vi "Auto Drive.vi"(7 "Distance":dbl format="%#_13g", 8 "error in (no error)":errorcluster, 9 "Angle":dbl format="%#_13g", 10 "Drive":T1[](array[typedef]), 11 "Swerve":T1[](array[typedef])) -> (0 "error IO":errorcluster)   [LabVIEW 2016]
uses:
  <vilib>/Rock Robotics/WPI/MotorControl/WPI_MotorControlDeviceRef.ctl
  <vilib>/Rock Robotics/WPI/MotorControl/WPI_MotorControlType.ctl
  <vilib>/Rock Robotics/SystemInterfaces/DIO/FPGA_DIOPWMChannel.ctl
  <vilib>/Rock Robotics/WPI/PWM/WPI_PWMDeadband.ctl
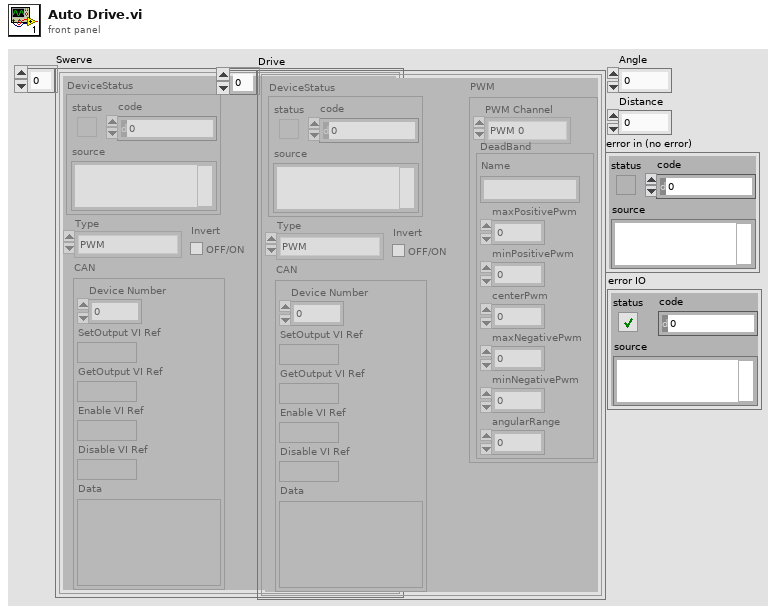
[diagram p1: front panel]
types:
  T1 = typedef "WPI_MotorControlDeviceRef.ctl" = cluster{"DeviceStatus":errorcluster, "Type":T2, "PWM":cluster{"PWM Channel":T3, "DeadBand":T4}, "CAN":cluster{"Device Number":u8, "SetOutput VI Ref":variant, "GetOutput VI Ref":variant, "Enable VI Ref":variant, "Disable VI Ref":variant, "Data":variant}, "Invert":bool}
  T2 = typedef "WPI_MotorControlType.ctl" = enum16{"PWM", "CAN"}
  T3 = typedef "FPGA_DIOPWMChannel.ctl" = enum8{"PWM 0", "PWM 1", "PWM 2", "PWM 3", "PWM 4", "PWM 5", "PWM 6", "PWM 7", "PWM 8", "PWM 9", "PWM MXP 0", "PWM MXP 1", "PWM MXP 2", "PWM MXP 3", "PWM MXP 4", "PWM MXP 5", "PWM MXP 6", "PWM MXP 7", "PWM MXP 8", "PWM MXP 9", "Invalid"}
  T4 = typedef "WPI_PWMDeadband.ctl" = cluster{"Name":string, "maxPositivePwm":i32, "minPositivePwm":i32, "centerPwm":i32, "maxNegativePwm":i32, "minNegativePwm":i32, "angularRange":u16}
  T5 = typedef "WPI_CANTalonSRX_GlobalStatus.ctl" = cluster{"Applied Throttle":dbl, "Module Enabled":bool, "CAN Error":errorcluster, "Closed Loop Error":dbl, "Forward Limit Switch Closed":bool, "Reverse Limit Switch Closed":bool, "Sensor Position":dbl, "Sensor Velocity":dbl, "Current":dbl, "Sticky Fault - Over Temp":bool, "Sticky Fault - Under Voltage":bool, "Sticky Fault - Forward Limit":bool, "Sticky Fault - Reverse Limit":bool, "Sticky Fault - Forward Soft Limit":bool, "Sticky Fault - Reverse Soft Limit":bool, "Brake is Enabled":bool, "Encoder Position":dbl, "Encoder Velocity":dbl, "Encoder Index Count":dbl, "Encoder A Pin State":bool, "Encoder B Pin State":bool, "Encoder Index Pin State":bool, "Analog In":dbl, "Analog In Velocity":dbl, "Temperature (C)":dbl, "Battery Voltage":dbl, "Control 5 Is Supported":bool, "Current Profile Slot Select":dbl, "Pos Div 8":bool, "Vel Div 4":bool, "Pulse Width Position":i32, "Pulse Width Velocity":i32, "Pulse Width Rise To Rise (us)":i32, "Pulse Width Rise To Fall (us)":i32, "Mot Prof Active Is Under Run":bool, "Mot Prof Active Has Under Run":bool, "Mot Prof Active Is Last":bool, "Mot Prof Active Velocity Only":bool, "Mot Prof Active Is Valid":bool, "Mot Prof Buffer Is Full":bool, "Mot Prof Active Profile Slot Select":i32, "Mot Prof NextID":i32, "Mot Prof Count":i32, "Mot Prof Active Velocity":dbl, "Mot Prof Active Position":dbl, "Mot Prof Output Enable":i32, "UsageFrame":u32, "Motion Magic Active Trajectory":cluster{"Velocity":dbl, "Position":dbl}}
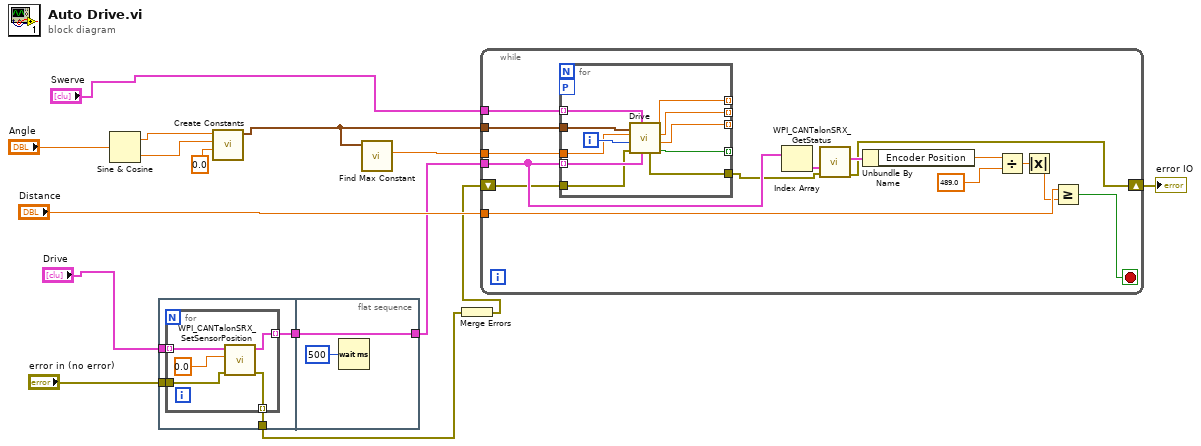
[diagram p0: block diagram]
diagram:
  n1 = Sine & Cosine(0:"Angle") -> (1:w13:dbl, 2:w12:dbl)
  n2 = flat-sequence {
    tunnel: "Drive" -> [w19]
    tunnel: [w18] -> w7
    tunnel: "error in (no error)" -> [w17]
    tunnel: [w16] -> w3
    tunnel: [w25] -> w5
    tunnel: w7 -> [w25]
    frame #0 {
      n3 = for {
        tunnel: w19 -> [w24] mode=indexing
        tunnel: [w22] -> w18 mode=indexing
        tunnel: w17 -> [w21]
        tunnel: [w20] -> w16 mode=indexing
        n4 = call <vilib>:"WPI_CANTalonSRX_SetSensorPosition.vi"("error in (no error)"=w21, "New Sensor Position"=0.0, "CAN Talon SRX Ref"=w24) -> ("error out"=w20:errorcluster, "CAN Talon SRX Ref"=w22:T1)  [unwired: 7 in]
      }
    }
    frame #1 {
      n5 = Wait (ms)(milliseconds to wait=u32 500) -> ()  [unwired: 1 out]
    }
  }
  n6 = call "Create Constants.vi"("Z"=0.0, "Y"=w12, "X"=w13) -> ("constants cluster"=w10:cluster{"a":dbl, "b":dbl, "c":dbl, "d":dbl})  [unwired: 8 in]
  n7 = call "Find Max Constant.vi"("constants in"=w10) -> ("Max or 1"=w9:dbl)  [unwired: 9 in, 1 out]
  n8 = Merge Errors(w3) -> (w2:errorcluster)
  n9 = while {
    tunnel: "Swerve" -> [w41]
    tunnel: w5 -> [w38]
    tunnel: w10 -> [w40]
    tunnel: w9 -> [w39]
    tunnel: "Distance" -> [w32]
    shift-right: [w27] -> w1
    shift-left: w2 -> [w29]
    stop <- w30 stop-if-true
    n10 = for {
      tunnel: w41 -> [w52] mode=indexing
      tunnel: [w50] -> _ mode=indexing
      tunnel: [w49] -> w28
      tunnel: w38 -> [w48] mode=indexing
      tunnel: [w47] -> _ mode=indexing
      tunnel: [w46] -> _ mode=indexing
      tunnel: [w45] -> _ mode=indexing
      workers-P: _ -> [_]
      tunnel: w40 -> [w44]
      tunnel: w39 -> [w43]
      tunnel: w29 -> [w42]
      i -> [w51]
      n11 = call "Drive.vi"("Wheel DevRef"=w48, "Swerve DevRef"=w52, "error in"=w42, "Index"=w51, "Max Speed or 1"=w43, "constants"=w44) -> ("Reverse?"=w50:bool, "Wheel Speed"=w45:dbl, "Setpoint"=w46:dbl, "Swerve Speed"=w47:dbl, "error out"=w49:errorcluster)  [unwired: 1 in]
    }
    n12 = Index Array(array=w38) -> (element=w37:T1)  [unwired: 1 in]
    n13 = call <vilib>:"WPI_CANTalonSRX_GetStatus.vi"("error in (no error)"=w28, "CAN Talon SRX Ref"=w37) -> ("error out"=w27:errorcluster, "Talon SRX Status"=w36:T5)  [unwired: 7 in, 1 out]
    n14 = Unbundle By Name(w36) -> ("Encoder Position"=w35:dbl)
    n15 = Divide(x=w35, y=489.0) -> (x/y=w33:dbl)
    n16 = Absolute Value(x=w33) -> (abs(x)=w31:dbl)
    n17 = Greater Or Equal?(x=w32, y=w31) -> (x >= y?=w30:bool)
  }
  "error IO" <- w1
